vi "ORB.vi"() -> ()   [LabVIEW 2009]
uses:
  Api/ORB/Orb_Global.vi
  Instance           4 11Saved   ORB .vi
panel:
  in  "PROCESS":string="ORB"
  in  "DebugLevel":i16
  out "Count":i32(knob)=100 scale=0.0..100.0
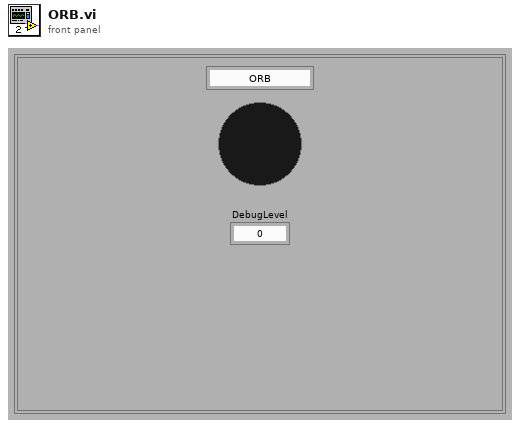
[diagram p1: front panel]
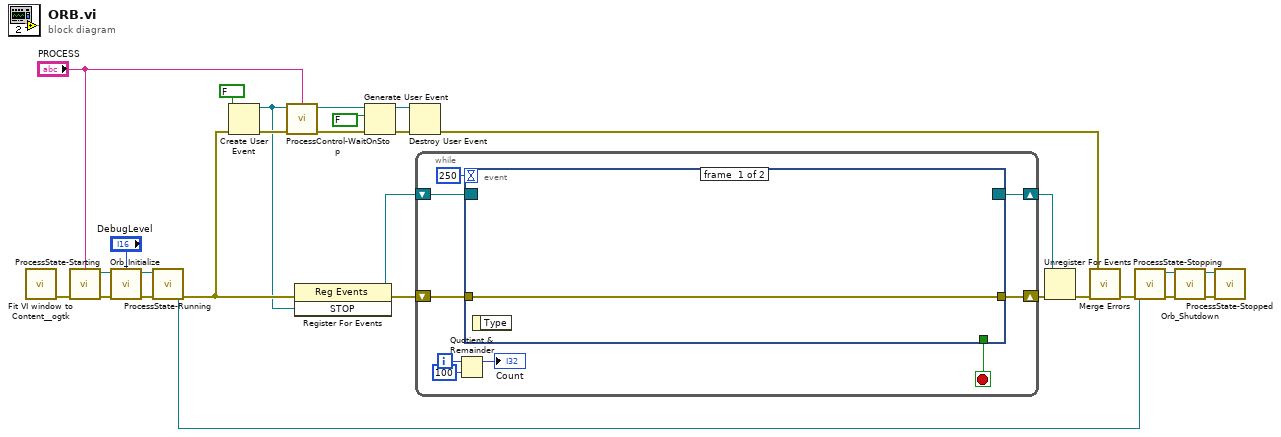
[diagram p0: block diagram]
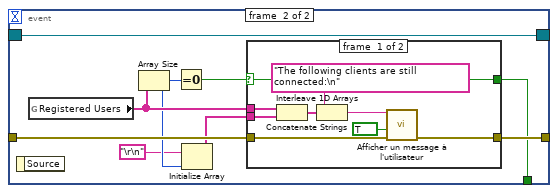
[diagram p2: hidden frame]
diagram:
  n1 = call <userlib>:"Fit VI window to Content__ogtk.vi"() -> ("error out"=w1:errorcluster)  [unwired: 3 in, 4 out]
  n2 = call "ProcessState-Starting.vi"("PROCESS"="PROCESS", "error in (no error)"=w1) -> ("ProcessStateNotifier"=w18:refnum<notifier>, "error in (no error)"=w20:errorcluster)  [unwired: 6 out]
  n3 = call "Orb_Initialize.vi"("traceLevel"="DebugLevel", "error in (no error)"=w20) -> ("error out"=w19:errorcluster)  [unwired: 7 out]
  n4 = call "ProcessState-Running.vi"("ProcessStateNotifier in"=w18, "error in (no error)"=w19) -> ("ProcessStateNotifier out"=w16:refnum<notifier>, "error out"=w9:errorcluster)  [unwired: 6 out]
  n5 = Create User Event(user event datatype=FALSE ("STOP"), error in=w9) -> (user event=w3:refnum<user-event>, error out=w11:errorcluster)
  n6 = call "ProcessControl-WaitOnStop.vi"("PROCESS"="PROCESS", "error out"=w11) -> ("error in"=w4:errorcluster)  [unwired: 7 out]
  n7 = register-events(error in=w9, w3) -> (reference out=w23:refnum<event-registration>, error out=w8:errorcluster)  [unwired: 1 in]
  n8 = Generate User Event(user event=w3, event data cluster=FALSE ("données d'événement"), error in=w4) -> (user event out=w12:refnum<user-event>, error out=w10:errorcluster)
  n9 = Destroy User Event(user event=w12, error in=w10) -> (error out=w5:errorcluster)
  n10 = while {
    shift-right: [w28] -> w22
    shift-left: w8 -> [w34]
    shift-right: [w26] -> w21
    shift-left: w23 -> [w27]
    i -> [w32]
    stop <- w29 stop-if-true
    n11 = Quotient & Remainder(x=w32, y=100) -> (x-y*floor(x/y)=→"Count":i32)  [unwired: 1 out]
    n12 = event shown="[1] <STOP>: User Event" {
      selector: w27 -> [_ w36]
      dyn-events: [_ w36] -> w26
      timeout: 250 -> [_ _]
      tunnel: w34 -> [w35 w44]
      tunnel: [_ w42] -> w29
      tunnel: [w35 w43] -> w28
      event #0 {
        n13 = event-data() -> ()  [unwired: 2 out]
      }
      event #1 {
        n14 = event-data() -> ()  [unwired: 2 out]
        n15 = global read "Orb_Global.vi" "Registered Users"() -> (w41:string[])
        n16 = Array Size(array=w41) -> (size(s)=w40:i32)
        n17 = Equal To 0?(x=w40) -> (x = 0?=w37:bool)
        n18 = Initialize Array("\r\n", w40) -> (w38:string[])
        n19 = case shown="True" w37 {
          selector: w37 -> [w51 w54]
          tunnel: w44 -> [w53 w55]
          tunnel: [w52 w55] -> w43
          tunnel: [w51 w54] -> w42
          tunnel: w41 -> [w49 _]
          tunnel: w38 -> [w48 _]
          frame #0 {
            n20 = Interleave 1D Arrays(w49, w48) -> (w47:string[])
            n21 = Concatenate Strings("The following clients are still connected:\n", w47) -> (w45:string)
            n22 = call "Afficher un message à l'utilisateur"("error in (no error)"=w53, "Enable"=TRUE, "Message"=w45) -> ("error out"=w52:errorcluster)  [unwired: 8 out]
          }
          frame #1 {
          }
        }
      }
    }
  }
  n23 = Unregister For Events(event registration refnum=w21, error in=w22) -> (error out=w7:errorcluster)
  n24 = call <vilib>:"Merge Errors.vi"("error in 3 (no error)"=w7, "error in 1 (no error)"=w5) -> ("error out"=w6:errorcluster)  [unwired: 2 in, 3 out]
  n25 = call "ProcessState-Stopping.vi"("ProcessStateNotifier in"=w16, "error in (no error)"=w6) -> ("ProcessStateNotifier out"=w14:refnum<notifier>, "error out"=w17:errorcluster)  [unwired: 6 out]
  n26 = call "Orb_Shutdown.vi"("error in (no error)"=w17) -> ("error out"=w15:errorcluster)  [unwired: 8 out]
  n27 = call "ProcessState-Stopped.vi"("ProcessStateNotifier in"=w14, "error in (no error)"=w15) -> ()  [unwired: 8 out]
